vi "controlNSteps.vi"(5 "set":bool=TRUE, 8 "error in":errorcluster, 9 "setnSteps in":i32=1, 10 "axis in":u8, 11 "connection ID":refnum<k5>) -> (0 "error out":errorcluster, 1 "setnSteps out":i32, 2 "axis out":u8, 3 "connection ID":refnum<k5>)   [LabVIEW 2016, in "AMC_VIs.lvlib"]
doc: "This function retrieves or triggers the number of steps on the selected axis and in the desired direction."
uses:
  AMC_VIs.lvlib
panel:
  in  "backward":bool
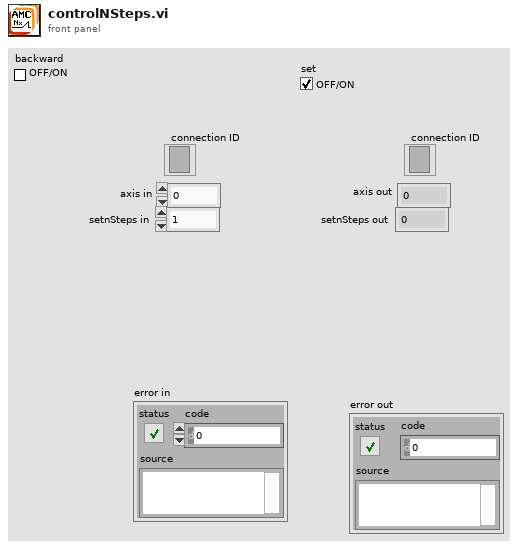
[diagram p1: front panel]
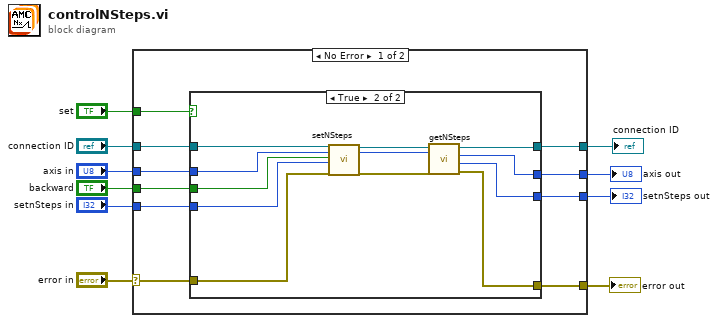
[diagram p0: block diagram]
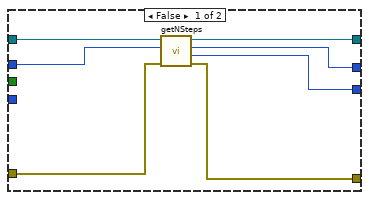
[diagram p2: hidden frame]
diagram:
  n1 = case shown="No Error" "error in" {
    selector: "error in" -> [w13 w40]
    tunnel: "axis in" -> [w17 w43]
    tunnel: [w12 w40] -> w9
    tunnel: [w15 w43] -> w8
    tunnel: "setnSteps in" -> [w16 w42]
    tunnel: [w18 w41] -> w6
    tunnel: "connection ID" -> [w19 w41]
    tunnel: [w14 w42] -> w3
    tunnel: "set" -> [w20 _]
    tunnel: "backward" -> [w11 _]
    frame No Error {
      n2 = case shown="True" w20 {
        tunnel: w19 -> [w27 w33]
        tunnel: [w26 w39] -> w18
        tunnel: w17 -> [w25 w32]
        tunnel: w16 -> [_ w31]
        tunnel: [w24 w38] -> w15
        tunnel: [w23 w37] -> w14
        tunnel: w13 -> [w22 w35]
        tunnel: [w21 w36] -> w12
        tunnel: w11 -> [_ w28]
        frame False {
          n3 = call "getNSteps.vi"("error in"=w22, "axis"=w25, "connection ID"=w27) -> ("error out"=w21:errorcluster, "nbrstep"=w23:i32, "axis_out"=w24:i32, "connection ID"=w26:refnum<k5>)  [unwired: 5 in]
        }
        frame True {
          n4 = call "setNSteps.vi"("connection ID"=w33, "axis"=w32, "backward"=w28, "step"=w31, "error in"=w35) -> ("connection ID"=w30:refnum<k5>, "axis_out"=w29:i32, "error out"=w34:errorcluster)  [unwired: 12 in]
          n5 = call "getNSteps.vi"("error in"=w34, "axis"=w29, "connection ID"=w30) -> ("error out"=w36:errorcluster, "nbrstep"=w37:i32, "axis_out"=w38:i32, "connection ID"=w39:refnum<k5>)  [unwired: 5 in]
        }
      }
    }
    frame Error {
    }
  }
  "error out" <- w9
  "axis out" <- w8
  "setnSteps out" <- w3
  "connection ID" <- w6
